vi "ULx Read (Analog Wfm 1Chan 1Samp).vi"(0 "task in":refnum<k24>, 9 "timeout":dbl=10.0 format="%_4g", 11 "error in":errorcluster) -> (4 "task out":refnum<k24>, 6 "data":waveform(dbl), 15 "error out":errorcluster)   [LabVIEW 2020]
doc: "Reads a waveform that contains a single sample from a task that contains a single analog input channel."
uses:
  C:/Users/William/Documents/LV 2020 builds/LeaktestDAQ/Source-v33/ULx_LV.dll
  ULx_LV.dll
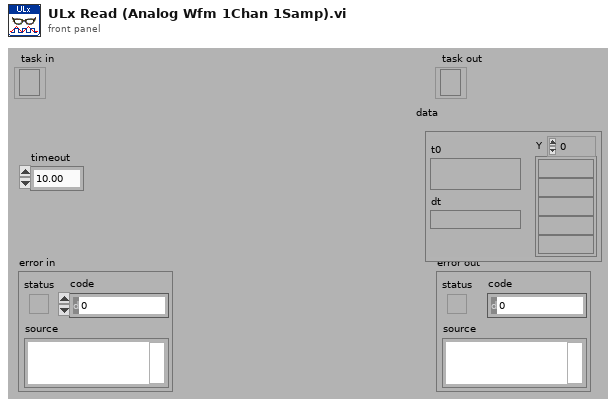
[diagram p1: front panel]
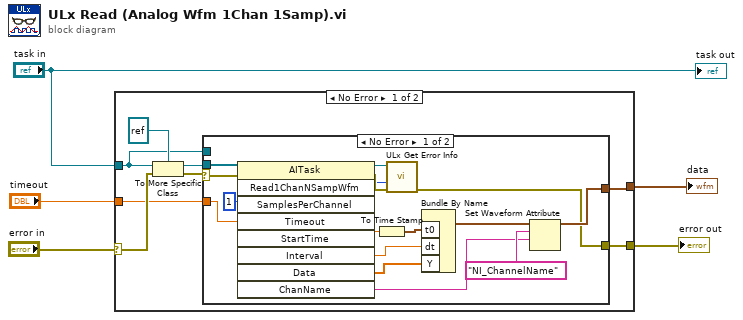
[diagram p0: block diagram]
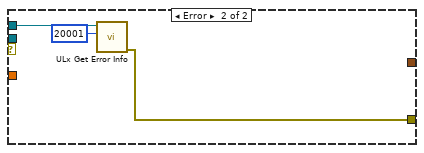
[diagram p2: hidden frame]
diagram:
  n1 = case shown="No Error" "error in" {
    selector: "error in" -> [w13 w33]
    tunnel: "task in" -> [w6 _]
    tunnel: "timeout" -> [w9 _]
    tunnel: [w7 _] -> w1
    tunnel: [w8 w33] -> w3
    frame No Error {
      n2 = To More Specific Class(target class=refnum<k24> refnum, reference=w6, error in=w13) -> (specific class reference=w10:refnum<k24>, error out=w11:errorcluster)
      n3 = case shown="No Error" w11 {
        selector: w11 -> [w28 _]
        tunnel: w10 -> [w29 _]
        tunnel: w9 -> [w19 _]
        tunnel: [w21 w30] -> w8
        tunnel: [w23 _] -> w7
        tunnel: w6 -> [_ w32]
        frame No Error {
          n4 = invoke class="AITask" method="Read1ChanNSampWfm"(reference=w29, error in=w28, "SamplesPerChannel"=1, "Timeout"=w19) -> (reference out=w27:refnum<k24>, error out=w22:errorcluster, "Read1ChanNSampWfm"=w20:i32, "StartTime"=w17:dbl, "Interval"=w16:dbl, "Data"=w15:dbl[], "ChanName"=w14:string)  [unwired: 5 in, 2 out]
          n5 = To Time Stamp(1:w17) -> (0:w26:timestamp)
          n6 = call "ULx Get Error Info.vi"("error in"=w22, "ErrorCode"=w20, "task in"=w27) -> ("error out"=w21:errorcluster)  [unwired: 8 in]
          n7 = Bundle By Name("t0"=w26, "dt"=w16, "Y"=w15) -> (w25:waveform(dbl))  [unwired: 1 in]
          n8 = Set Waveform Attribute(5:w14, 6:"NI_ChannelName", 7:w25) -> (3:w23:waveform(dbl))  [unwired: 1 in, 2 out]
        }
        frame Error {
          n9 = call "ULx Get Error Info.vi"("ErrorCode"=20001, "task in"=w32) -> ("error out"=w30:errorcluster)  [unwired: 9 in]
        }
      }
    }
    frame Error {
    }
  }
  "error out" <- w3
  "data" <- w1
  "task out" <- "task in"
